vi "Increment Next Bind.vi"(11 "SQL Statement in":refnum<class "SQL Statement.lvclass">) -> (2 "Paramter #":i32, 3 "SQL Statement out":refnum<class "SQL Statement.lvclass">)   [LabVIEW 2011]
uses:
  SQL Statement.lvclass
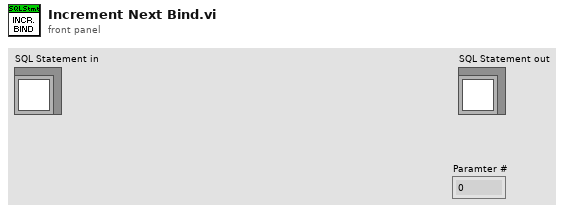
[diagram p1: front panel]
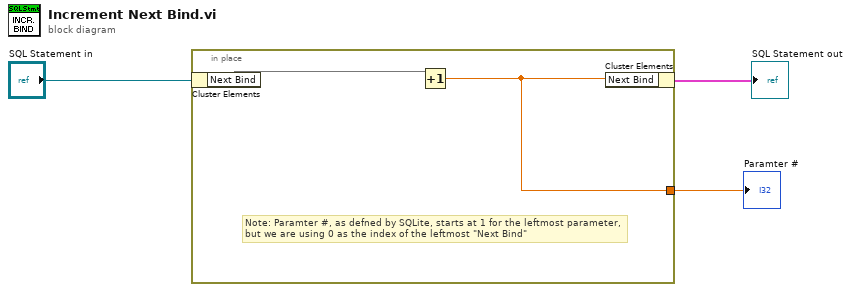
[diagram p0: block diagram]
diagram:
  n1 = in-place {
    in-place-border: [w4] -> w1
    # "Note: Paramter #, as defned by SQLite, starts at 1 for the leftmost parameter,\nbut we are using 0 as the index of the leftmost \"Next Bind\""
    n2 = in-place-cluster #1("SQL Statement in") -> ("Next Bind"=w5)
    n3 = Increment(x=w5) -> (x+1=w4:dbl)
    n4 = in-place-cluster #1("Next Bind"=w4) -> (→"SQL Statement out":cluster{})
  }
  "Paramter #" <- w1
